vi "LabVIEW Basics #5.vi"() -> ()   [LabVIEW 2021]
uses:
  <vilib>/picture/picture.llb/imagedata.ctl
panel:
  out "ping":bool
  out "Degrees":dbl format="%#_3f"
  out "Distance":dbl caption="CM" format="%#_2g"
  out "2D Picture":picture
  in  "Stop":bool
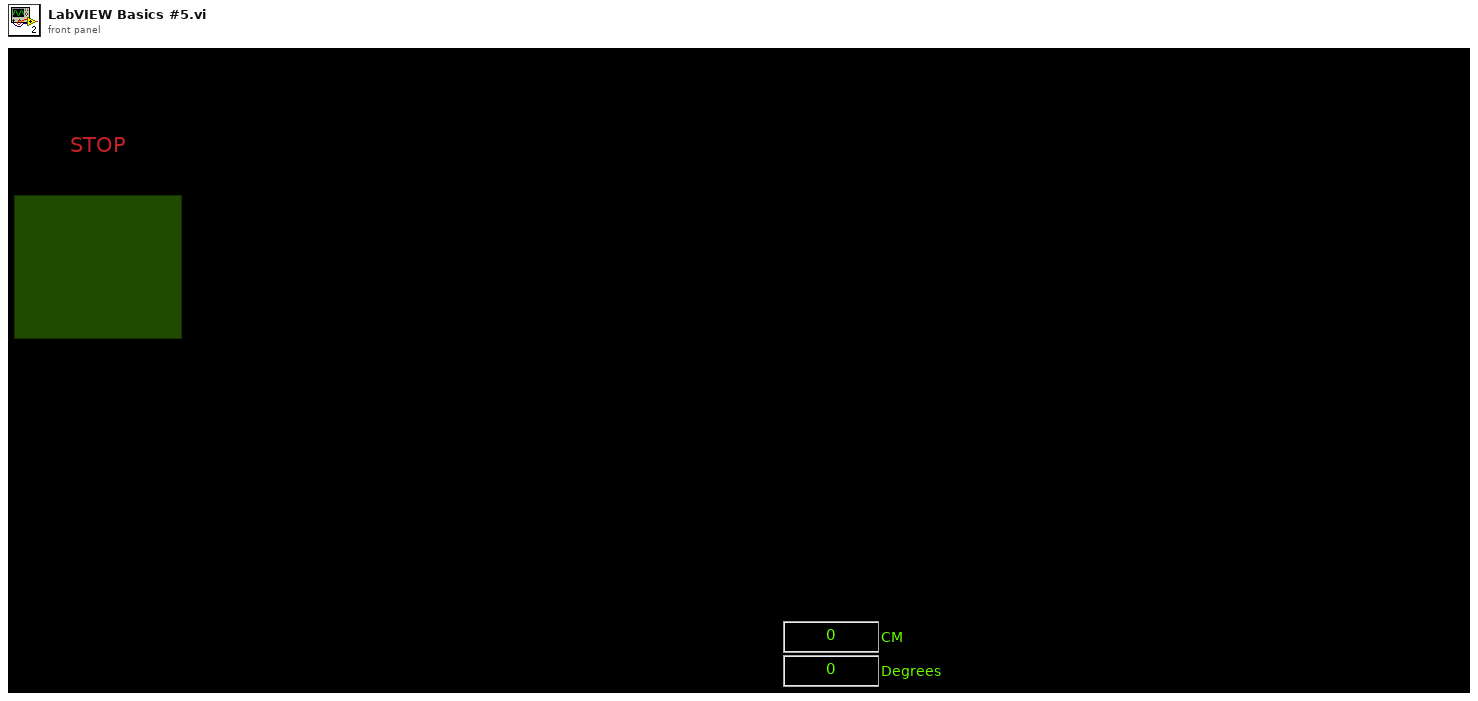
[diagram p1: front panel]
types:
  T1 = typedef "imagedata.ctl" = cluster{"image type":i32, "image depth":i32, "image":u8[], "mask":u8[], "colors":u32[], "Rectangle":cluster{"left":i16, "top":i16, "right":i16, "bottom":i16}}
  T2 = cluster{"maximum":dbl, "minimum":dbl, "clip to min":bool, "log?(F)":bool, "grid color":u32, "plot color":u32, "format and precision":cluster{"format":enum8{"Decimal", "Scientific", "Engineering", "Binary", "Octal", "Hex"}, "precision":u8}, "visible section":u16}
  T3 = typedef "LVBoundsTypeDef.ctl" = cluster{"Width":u32, "Height":u32}
  T4 = cluster{"pixel center":cluster{"x":i16, "y":i16}, "scale factors":cluster{"a":dbl, "b":dbl, "log?":bool}, "grid color":u32, "start angle":dbl, "end angle":dbl, "tick length":i16, "pixel radius":i32}
  T5 = cluster{"Distance (cm)":dbl, "Angle (Deg)":dbl}[]
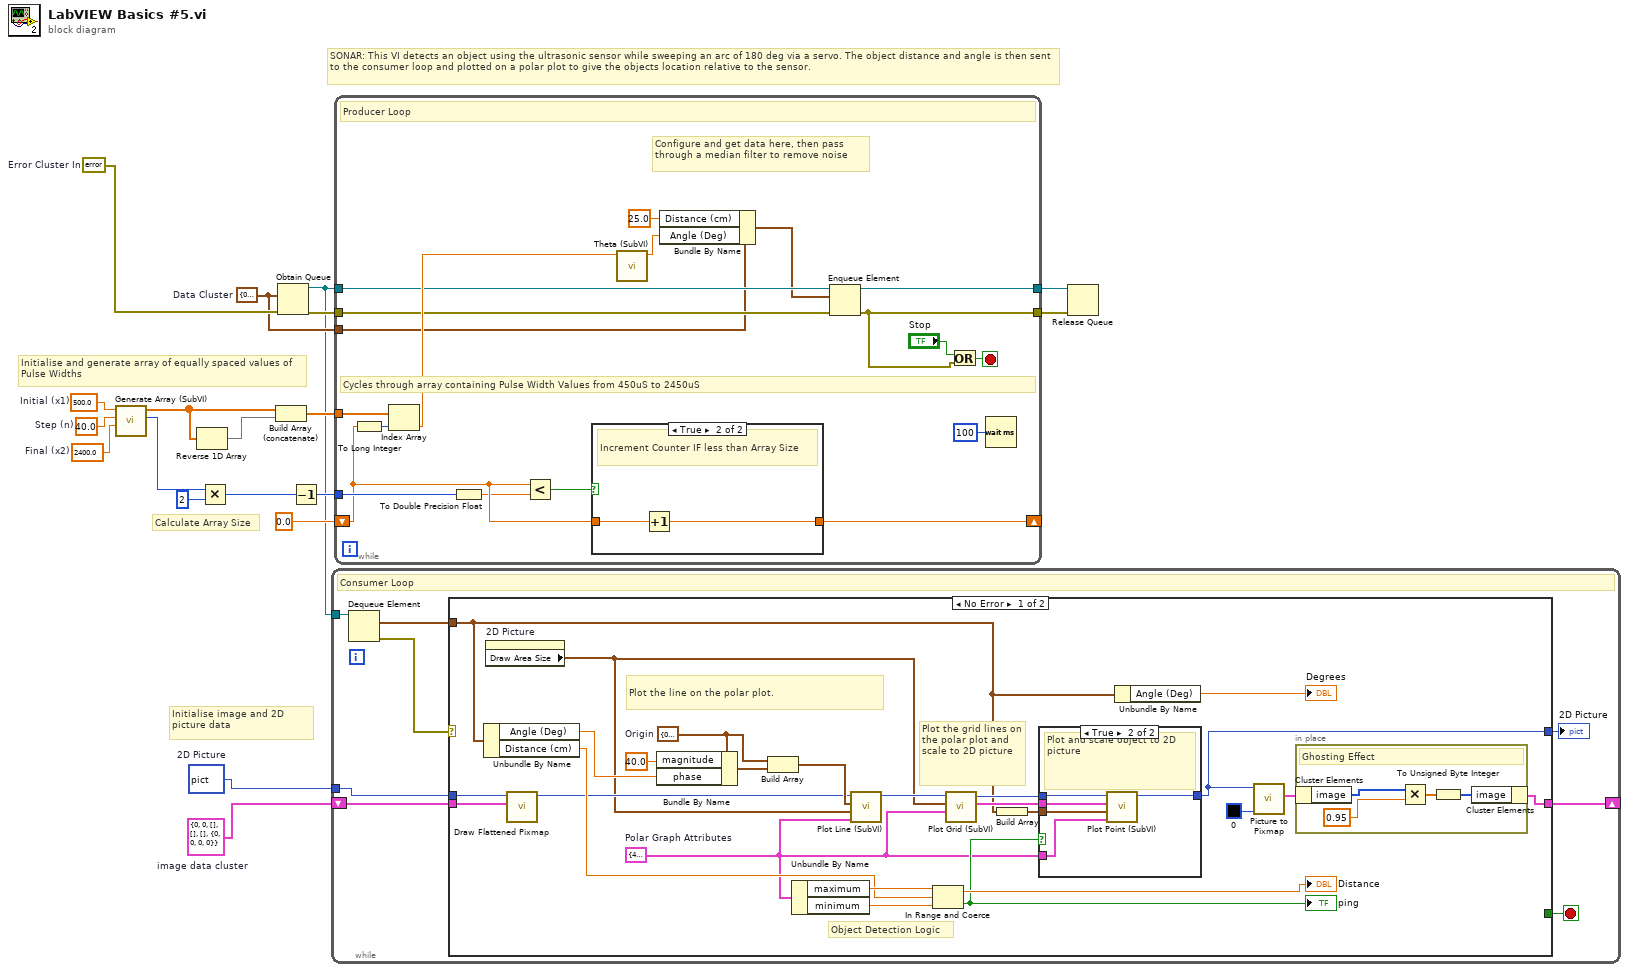
[diagram p0: block diagram]
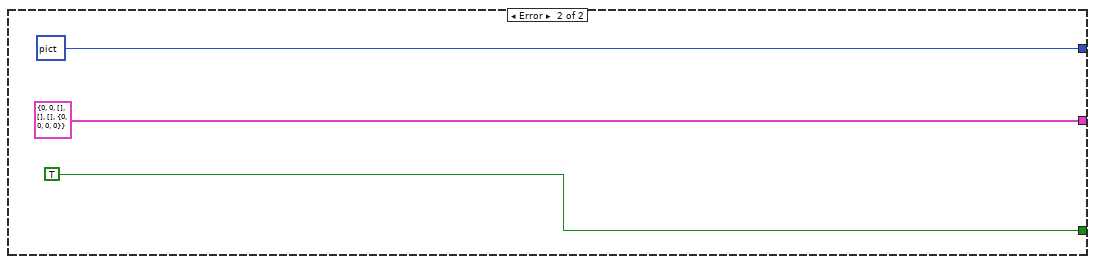
[diagram p3: hidden frame]
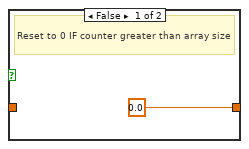
[diagram p4: hidden frame]
diagram:
  w1 = T1 {"image type"=0, "image depth"=0, "image"=[], "mask"=[], "colors"=[], "Rectangle"={"left"=0, "top"=0, "right"=0, "bottom"=0}}  # image data cluster
  w2 = picture data[5B]  # 2D Picture
  w4 = cluster{"Distance (cm)":dbl, "Angle (Deg)":dbl} {"Distance (cm)"=0.0, "Angle (Deg)"=0.0}  # Data Cluster
  w17 = 2400.0  # Final (x2)
  w16 = 40.0  # Step (n)
  w15 = 500.0  # Initial (x1)
  w7 = errorcluster {"status"=FALSE, "code"=0, "source"=""}  # Error Cluster In
  # "Initialise image and 2D picture data"
  # "Calculate Array Size"
  # "Initialise and generate array of equally spaced values of Pulse Widths"
  # "SONAR: This VI detects an object using the ultrasonic sensor while sweeping an arc of 180 deg via a servo. The object distance and angle is then sent to the consumer loop and plotted on a polar plot to give the objects location relative to the sensor."
  n1 = call "Generate Array (SubVI).vi"("Final"=w17, "Step"=w16, "Initial"=w15) -> ("Array size"=w10:i32, "Array out"=w13:dbl[])  [unwired: 6 in, 1 out]
  n2 = Reverse 1D Array(array=w13) -> (reversed array=w12:dbl[])
  n3 = Multiply(x=w10, y=2) -> (x*y=w11:i32)
  n4 = Build Array (concatenate)(w13, w12) -> (w14:dbl[])
  n5 = Obtain Queue(element data type=w4, error in (no error)=w7) -> (queue out=w3:refnum<queue>, error out=w8:errorcluster)  [unwired: 3 in, 1 out]
  n6 = Decrement(x=w11) -> (x-1=w18:i32)
  n7 = while {
    tunnel: w3 -> [w20]
    tunnel: w2 -> [w24]
    shift-right: [w21] -> _
    shift-left: w1 -> [w23]
    stop <- w25 stop-if-true
    # "Consumer Loop"
    n8 = Dequeue Element(queue=w20) -> (element=w26:cluster{"Distance (cm)":dbl, "Angle (Deg)":dbl}, error out=w27:errorcluster)  [unwired: 2 in, 2 out]
    n9 = case shown="No Error" w27 {
      tunnel: w26 -> [w35 _]
      tunnel: [_ TRUE] -> w25
      tunnel: w24 -> [w52 _]
      tunnel: w23 -> [w51 _]
      tunnel: [w47 picture data[5B] ("new picture")] -> w22
      tunnel: [w50 T1 {"image type"=0, "image depth"=0, "image"=[], "mask"=[], "colors"=[], "Rectangle"={"left"=0, "top"=0, "right"=0, "bottom"=0}} ("image data")] -> w21
      frame No Error {
        w33 = T2 {"maximum"=40.0, "minimum"=2.0, "clip to min"=TRUE, "log?(F)"=FALSE, "grid color"=9868950, "plot color"=65280, "format and precision"={"format"=enum."Decimal", "precision"=0}, "visible section"=4}  # Polar Graph Attributes
        w29 = cluster{"magnitude":dbl, "phase":dbl} {"magnitude"=0.0, "phase"=0.0}  # Origin
        # "Object Detection Logic"
        # "Plot the line on the polar plot."
        # "Plot the grid lines on the polar plot and scale to 2D picture"
        n10 = Unbundle By Name(w35) -> ("Angle (Deg)"=w40:dbl, "Distance (cm)"=w41:dbl)
        n11 = property on="2D Picture" class="Pict"() -> ("Draw Area Size"=w37:T3)  [unwired: 2 in, 2 out]
        n12 = call <vilib>:"Draw Flattened Pixmap.vi"("image data"=w51, "picture"=w52) -> ("new picture"=w38:picture)  [unwired: 7 in]
        n13 = Bundle By Name(cluster=w29, "magnitude"=40.0, "phase"=w40) -> (w28:cluster{"magnitude":dbl, "phase":dbl})
        n14 = Build Array(w29, w28) -> (w48:cluster{"magnitude":dbl, "phase":dbl}[])
        n15 = Unbundle By Name(w33) -> ("maximum"=w43:dbl, "minimum"=w42:dbl)
        n16 = call "Plot Line (SubVI).vi"("Polar Graph Attributes"=w33, "Draw Area Size"=w37, "Polar Array"=w48, "new picture in"=w38) -> ("new picture out"=w49:picture)  [unwired: 7 in]
        n17 = In Range and Coerce(upper limit=w43, x=w41, lower limit=w42) -> (coerced(x)=→"Distance":dbl, In Range?=w39:bool)
        "ping" <- w39
        n18 = call "Plot Grid (SubVI).vi"("Polar Graph Attributes"=w33, "Draw Area Size"=w37, "new picture in"=w49) -> ("grid measurements"=w45:T4, "new picture out"=w46:picture)  [unwired: 7 in]
        n19 = Build Array(w35) -> (w36:T5)
        n20 = case shown="True" w39 {
          tunnel: w36 -> [_ w58]
          tunnel: [w57 w62] -> w47
          tunnel: w46 -> [w57 w60]
          tunnel: w45 -> [_ w59]
          tunnel: w33 -> [_ w61]
          frame False {
            # "Nothing Detected"
          }
          frame True {
            # "Plot and scale object to 2D picture"
            n21 = call "Plot Point (SubVI).vi"("Polar Graph Attributes"=w61, "Array"=w58, "grid measurements"=w59, "new picture in"=w60) -> ("new picture"=w62:picture)  [unwired: 7 in]
          }
        }
        n22 = Unbundle By Name(w35) -> ("Angle (Deg)"=→"Degrees":dbl)
        n23 = call <vilib>:"Picture to Pixmap.vi"("Background Color"=u32 0, "picture"=w47) -> ("image data"=w32:T1)  [unwired: 8 in, 1 out]
        n24 = in-place {
          # "Ghosting Effect"
          n25 = in-place-cluster #1(w32) -> ("image"=w56:u8[])
          n26 = Multiply(x=w56, y=0.95) -> (x*y=w54:dbl[])
          n27 = To Unsigned Byte Integer(number=w54) -> (unsigned 8bit integer=w53:u8[])
          n28 = in-place-cluster #1("image"=w53) -> (w50:T1)
        }
      }
      frame Error {
      }
    }
    "2D Picture" <- w22
  }
  n29 = while {
    tunnel: w14 -> [w83]
    shift-right: [w79] -> _
    shift-left: 0.0 -> [w81]
    tunnel: w18 -> [w82]
    tunnel: w4 -> [w73]
    tunnel: w8 -> [w77]
    tunnel: [w67] -> w5
    tunnel: w3 -> [w76]
    tunnel: [w75] -> w6
    stop <- w84 stop-if-true
    # "Configure and get data here, then pass through a median filter to remove noise"
    # "Cycles through array containing Pulse Width Values from 450uS to 2450uS"
    # "Producer Loop"
    n30 = To Long Integer(number=w81) -> (32bit integer=w69:i32)
    n31 = Index Array "Index Array"(array=w83, index=w69) -> (element=w78:dbl)
    n32 = To Double Precision Float(number=w82) -> (double precision float=w68:dbl)
    n33 = Less?(x=w81, y=w68) -> (x < y?=w80:bool)
    n34 = case shown="True" w80 {
      tunnel: [0.0 w87] -> w79
      tunnel: w81 -> [_ w86]
      frame False {
        # "Reset to 0 IF counter greater than array size"
      }
      frame True {
        # "Increment Counter IF less than Array Size"
        n35 = Increment(x=w86) -> (x+1=w87:dbl)
      }
    }
    n36 = call "Theta (SubVI).vi"("PWM"=w78) -> ("Theta"=w74:dbl)  [unwired: 9 in, 1 out]
    n37 = Bundle By Name(cluster=w73, "Distance (cm)"=25.0, "Angle (Deg)"=w74) -> (w72:cluster{"Distance (cm)":dbl, "Angle (Deg)":dbl})
    n38 = Enqueue Element(queue=w76, element=w72, error in (no error)=w77) -> (queue out=w75:refnum<queue>, error out=w67:errorcluster)  [unwired: 1 in, 1 out]
    n39 = Or(x="Stop", y=w67) -> (x .or. y?=w84:bool)
    n40 = Wait (ms)(milliseconds to wait=u32 100 ("Slide")) -> ()  [unwired: 1 out]
  }
  n41 = Release Queue(queue=w6, error in (no error)=w5) -> ()  [unwired: 1 in, 3 out]
